vi "from_node_ids.vi"(5 "edge type":refnum<class "Edge.lvclass">, 9 "sink-id":refnum<class "ID.lvclass">, 10 "source-id":refnum<class "ID.lvclass">) -> (3 "new edge":refnum<class "Edge.lvclass">)   [LabVIEW 2020, in "graph.lvlib" / "Edge.lvclass"]
uses:
  Edge.lvclass
  ID/ID.lvclass
  Edge.lvclass/Edge.ctl
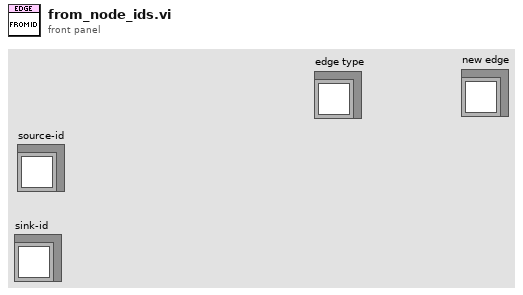
[diagram p1: front panel]
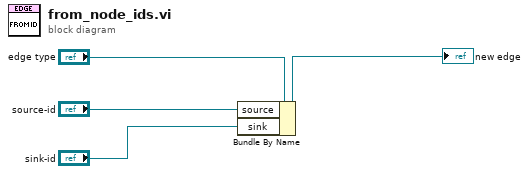
[diagram p0: block diagram]
diagram:
  n1 = Bundle By Name(cluster="edge type", "source"="source-id", "sink"="sink-id") -> (→"new edge":refnum<class "Edge.lvclass">)
